vi "ADC_GetDataCh.vi"(8 "error in (no error)":errorcluster, 10 "wData":i16, 11 "wCh":i16) -> (0 "error out":errorcluster, 2 "wData out":i16, 3 "function return":i16)   [LabVIEW 2013, in "HS3AcquireData.lvlib"]
doc: "Description: This routine transfers the measured data of one channel from theacquisition memory in the hardware via the DLL into the memory in the application. The measured data is returned in binary values. A value of 0 corresponds to -Sensitivity, 32768 corresponds to 0 and 65535 to +Sensitivity in Volts. wData is an array. The caller must ensure that there is enough space in the array to contain the data. Therefore the size of the array in bytes must be at least\nRecordLength * sizeof( word )\n\nInput: wCh Indicates from which channel the data has to be\nretrieved\nOutput: wData The array to which the measured data of the\nrequested channel should be passed.\nReturn value E_NO_ERRORS | E_NO_HARDWARE\n\nFunction prototype: word ADC_GetDataCh( word wCh, word *wData )\n\nshort int ADC_GetDataCh ( short int wCh, short int *wData );"
uses:
  HS3AcquireData.lvlib
  hs3.dll
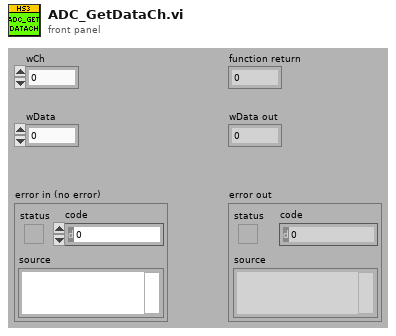
[diagram p1: front panel]
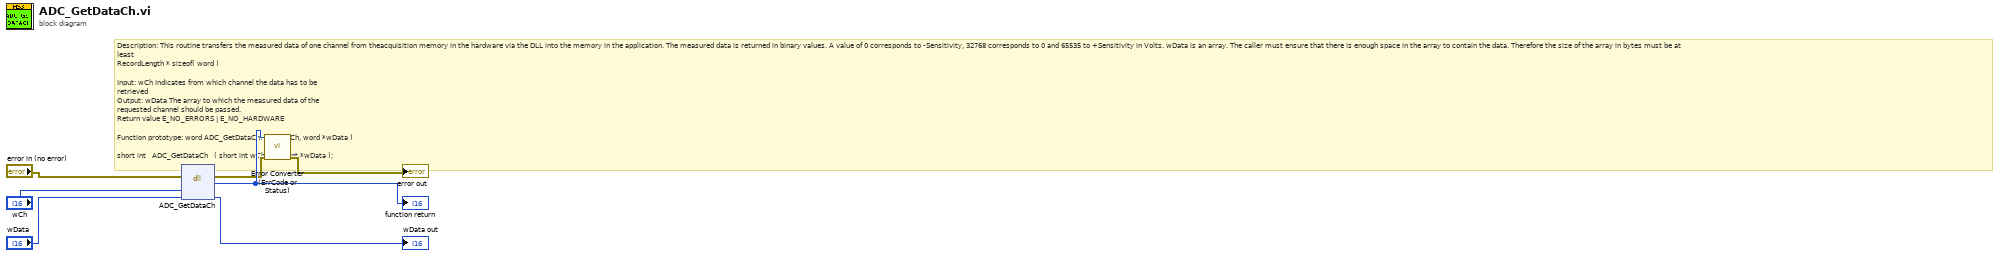
[diagram p0: block diagram]
diagram:
  # "Description: This routine transfers the measured data of one channel from theacquisition memory in the hardware via the DLL into the memory in the application. The measured data is returned in binary values. A value of 0 corresponds to -Sensitivity, 32768 corresponds to 0 and 65535 to +Sensitivity in Volts. wData is an array. The caller must ensure that there is enough space in the array to contain the data. Therefore the size of the array in bytes must be at least\nRecordLength * sizeof( word )\n\nInput: wCh Indicates from which channel the data has to be\nretrieved\nOutput: wData The array to which the measured data of the\nrequested channel should be passed.\nReturn value E_NO_ERRORS | E_NO_HARDWARE\n\nFunction prototype: word ADC_GetDataCh( word wCh, word *wData )\n\nshort int \t\tADC_GetDataCh\t\t\t( short int wCh, short int *wData );"
  n1 = dll-call lib="C:/Documents and Settings/admin/Pulpit/HS3 LabViewLib/HS3_WRAPPER/AcquireData/hs3.*" fn="ADC_GetDataCh"(error in="error in (no error)", "wCh"="wCh", "wData"="wData") -> (error out=w2:errorcluster, w7:i16, "wData"=→"wData out":i16)  [unwired: 3 in, 1 out]
  "function return" <- w7
  n2 = call "Error Converter (ErrCode or Status).vi"("error in (no error)"=w2, "error code"=w7) -> ("error out"=→"error out":errorcluster)  [unwired: 9 in]
